vi "PicoScope2000aExampleAWG.vi"() -> ()   [LabVIEW 2010]
uses:
  ps2000a.dll
panel:
  in  "error in (no error)":errorcluster
  in  "Standard Waveform Settings":T1={"Start Frequency"=1000.0, "Stop Frequency"=1000.0, "Increment"=0.0, "Dwell Time (seconds)"=0.0} {"Stop Frequency" min=0.03 max=1000000.0; "Start Frequency" min=0.03 max=1000000.0}
  in  "Arbitrary Waveform Settings":T2 {"Index Mode" items=["Single", "Dual", "Quad"]}
  in  "Software \nTrigger":bool
  in  "Stop S/W \nTrigger":bool
  out "Arbitrary\nWaveform Graph":i16[](graph)
  in  "Update":bool
  in  "stop":bool
  in  "General AWG Settings":T3={"Peak-to-Peak Voltage (microvolts)"=1000000, "Offset Voltage (microvolts)"=0, "Wave Type"=0, "Sweep Type"=0, "Shots"=0, "Sweeps"=0, "Trigger Type"=0, "Trigger Source"=0, "Ext. Threshold (ADC count)"=0, "White Noise"=FALSE} {"Trigger Source" items=["None", "Scope Trigger", "Aux. In", "Ext. In", "Software Trigger"]; "Trigger Type" items=["Rising", "Falling", "Gate High", "Gate Low"]; "Sweep Type" items=["Up", "Down", "Up-Down", "Down-Up"]; "Wave Type" items=["Sine"=0, "Square"=1, "Triangle"=2, "Ramp Up"=3, "Ramp Down"=4, "DC"=8, "Arbitrary"=6]}
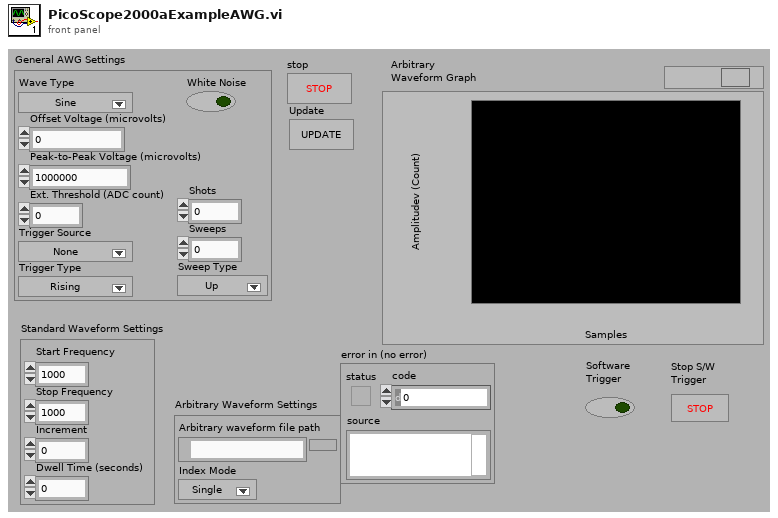
[diagram p1: front panel]
types:
  T1 = cluster{"Start Frequency":dbl, "Stop Frequency":dbl, "Increment":dbl, "Dwell Time (seconds)":dbl}
  T2 = cluster{"Arbirary waveform file path":path, "Index Mode":u32}
  T3 = cluster{"Peak-to-Peak Voltage (microvolts)":u32, "Offset Voltage (microvolts)":i32, "Wave Type":i16, "Sweep Type":i32, "Shots":u32, "Sweeps":u32, "Trigger Type":i32, "Trigger Source":i32, "Ext. Threshold (ADC count)":i16, "White Noise":bool}
  T4 = cluster{"Driver Version":string, "USB Version":string, "Hardware":string, "Variant":string, "Batch and Serial":string, "Cal Date":string, "Kernel Version":string, "Digital HW Version":string, "Analogue HW Version":string, "Firmware 1":string, "Firmware 2":string, "MSO":bool, "Number of Channels":i16}
  T5 = cluster{"status":bool, "code":u32, "source":string}
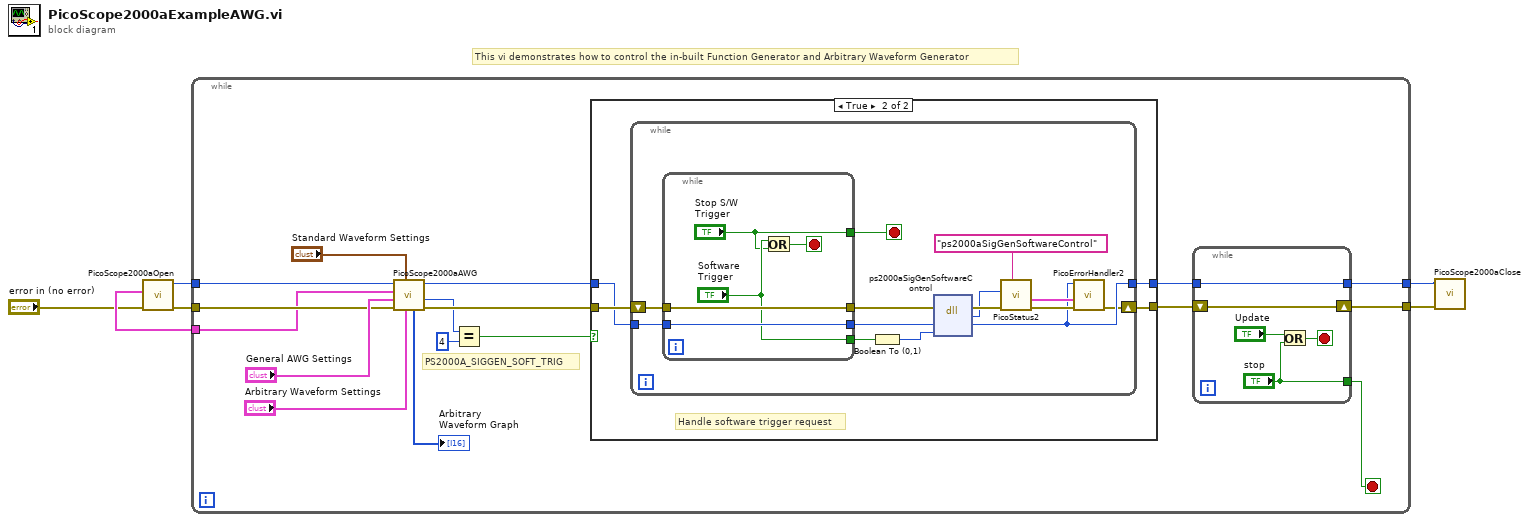
[diagram p0: block diagram]
diagram:
  # "This vi demonstrates how to control the in-built Function Generator and Arbitrary Waveform Generator"
  n1 = call "PicoScope2000aOpen.vi"("error in (no error)"="error in (no error)") -> ("error out"=w5:errorcluster, "Device Info"=w4:T4, "handle"=w6:i16)  [unwired: 5 in, 3 out]
  n2 = while {
    tunnel: w6 -> [w12]
    tunnel: w5 -> [w10]
    tunnel: w4 -> [w8]
    tunnel: [w13] -> w2
    tunnel: [w14] -> w1
    stop <- w22 stop-if-true
    # "PS2000A_SIGGEN_SOFT_TRIG"
    n3 = call "PicoScope2000aAWG.vi"("Arbitrary Waveform Settings"="Arbitrary Waveform Settings", "Standard Waveform Settings"="Standard Waveform Settings", "error in"=w10, "General AWG Settings"="General AWG Settings", "Device Info"=w8, "Handle In"=w12) -> ("error out"=w9:errorcluster, "triggerSource"=w7:i32, "Handle Out"=w11:i16, "Arbitrary\nWaveform Graph"=→"Arbitrary\nWaveform Graph":i16[])  [unwired: 2 in]
    n4 = Equal?(x=w7, y=4) -> (x = y?=w20:bool)
    n5 = case shown="True" w20 {
      tunnel: w9 -> [w25 w29]
      tunnel: w11 -> [w24 w28]
      tunnel: [w25 w26] -> w16
      tunnel: [w24 w27] -> w15
      frame False {
      }
      frame True {
        # "Handle software trigger request"
        n6 = while {
          tunnel: w28 -> [w41]
          tunnel: [w31] -> w27
          shift-right: [w30] -> w26
          shift-left: w29 -> [w42]
          stop <- w37 stop-if-true
          n7 = while {
            tunnel: [w48] -> w43
            tunnel: w42 -> [w48]
            tunnel: ["Software \nTrigger"] -> w39
            tunnel: w41 -> [w47]
            tunnel: [w47] -> w40
            tunnel: ["Stop S/W \nTrigger"] -> w37
            stop <- w44 stop-if-true
            n8 = Or(x="Software \nTrigger", y="Stop S/W \nTrigger") -> (x .or. y?=w44:bool)
          }
          n9 = Boolean To (0,1)(Boolean=w39) -> (0, 1=w38:i16)
          n10 = dll-call lib="ps2000a.dll" fn="ps2000aSigGenSoftwareControl"(error in=w43, "handle"=w40, "state"=w38) -> (error out=w34:errorcluster, "PICO_STATUS"=w33:u32, "handle"=w31:i16)  [unwired: 3 in, 1 out]
          n11 = call "PicoStatus2.vi"("PICO source"="ps2000aSigGenSoftwareControl" ("source"), "Error in"=w34, "PICO STATUS"=w33) -> ("error out"=w36:errorcluster, "PICO_STATUS out"=w35:T5)  [unwired: 5 in]
          n12 = call "PicoErrorHandler2.vi"("error in (no error)"=w36, "PICO_STATUS in"=w35, "handle In"=w31) -> ("error out"=w30:errorcluster)  [unwired: 8 in]
        }
      }
    }
    n13 = while {
      tunnel: ["stop"] -> w22
      tunnel: w15 -> [w50]
      tunnel: [w50] -> w14
      shift-right: [w49] -> w13
      shift-left: w16 -> [w49]
      stop <- w53 stop-if-true
      n14 = Or(x="Update", y="stop") -> (x .or. y?=w53:bool)
    }
  }
  n15 = call "PicoScope2000aClose.vi"("error in (no error)"=w2, "handle in"=w1) -> ()  [unwired: 8 in, 2 out]
